vi "Open All Relays_DAQmx_CreateVirtualChannel.vi"(0 "Device/Ports/Lines":string="Dev1/port0/line0,Dev1/port0/line1,Dev1/port0/line2,Dev1/port0/line3,Dev1/port0/line4,Dev1/port0/line5,Dev1/port0/line6,Dev1/port0/line7,\nDev1/port0/line8,Dev1/port0/line9,Dev1/port0/line10,Dev1/port0/line11,Dev1/port0/line12,Dev1/port0/line13,Dev1/port0/line14,Dev1/port0/line15,\nDev1/port0/line16,Dev1/port0/line17,Dev1/port0/line18,Dev1/port0/line19,Dev1/port0/line20,Dev1/port0/line21,\nDev1/port0/line22,Dev1/port0/line23,Dev1/port0/line24,Dev1/port0/line25,\nDev1/port0/line26,Dev1/port0/line27,Dev1/port0/line28,Dev1/port0/line29,Dev1/port0/line30,Dev1/port0/line31,\nDev1/port1/line0,Dev1/port1/line1,Dev1/port1/line2,Dev1/port1/line3,Dev1/port1/line4,Dev1/port1/line5,Dev1/port1/line6,Dev1/port1/line7,\nDev1/port2/line0,Dev1/port2/line1,Dev1/port2/line2,Dev1/port2/line3,Dev1/port2/line4,Dev1/port2/line5,Dev1/port2/line6,Dev1/port2/line7\n", 2 "Boolean":bool, 3 "error in":errorcluster) -> (7 "Array":bool[](array[boolean]), 10 "error out":errorcluster)   [LabVIEW 2015]
uses:
  <vilib>/DAQmx/write.llb/DAQmx Write (Digital 1D Bool 1Chan 1Samp).vi
  <vilib>/DAQmx/create/channels.llb/DAQmx Create Channel (DO-Digital Output).vi
  <vilib>/DAQmx/miscellaneous.llb/DAQmx Fill In Error Info.vi
panel:
  # "False means open relay"
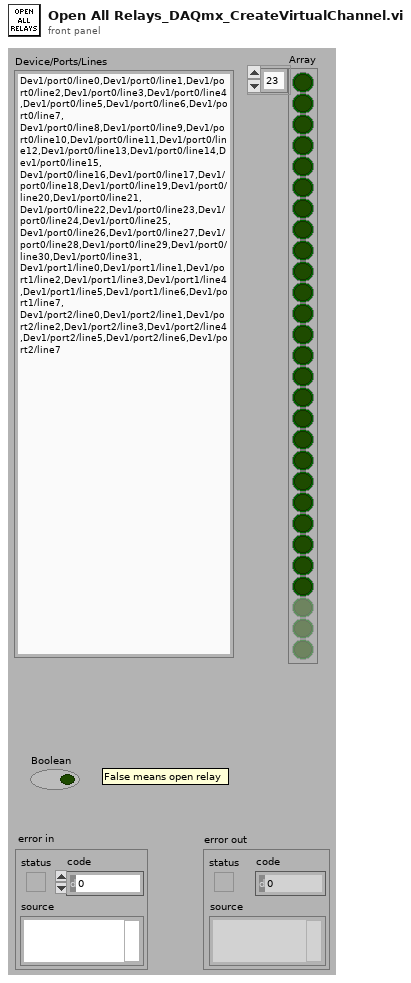
[diagram p1: front panel]
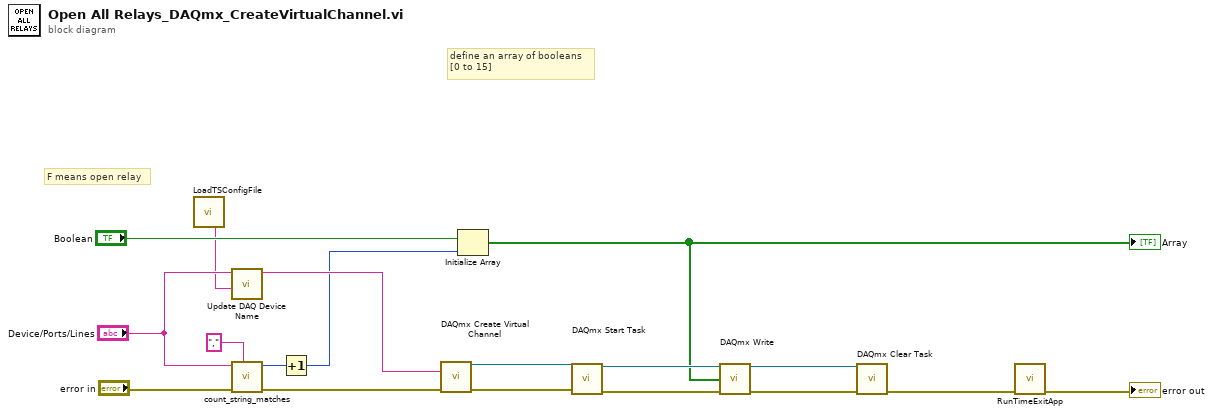
[diagram p0: block diagram]
diagram:
  # "define an array of booleans\n[0 to 15]"
  # "F means open relay"
  n1 = call "LoadTSConfigFile.vi"() -> ("DAQDevice"=w1:string)  [unwired: 5 in, 10 out]
  n2 = call "Update DAQ Device Name.vi"("Device Name"=w1, "Lines in (String)"="Device/Ports/Lines") -> ("Lines out (DAQmx Physical Channels)"=w10:tag)  [unwired: 9 in]
  n3 = call "count_string_matches.vi"("String"="Device/Ports/Lines", "error in (no error)"="error in", "String to Match"=",") -> ("Number of matches"=w18:i32, "error out"=w8:errorcluster)  [unwired: 6 in]
  n4 = Increment(x=w18) -> (x+1=w5:i32)
  n5 = call-poly <vilib>:"DAQmx Create Virtual Channel.vi"("lines"=w10, "error in"=w8) -> ("task out"=w15:refnum<k21>, "error out"=w16:errorcluster)  [unwired: 12 in]
  n6 = Initialize Array("Boolean", w5) -> (w4:bool[])
  "Array" <- w4
  n7 = call <vilib>:"DAQmx Start Task.vi"("task/channels in"=w15, "error in"=w16) -> ("task out"=w14:refnum<k21>, "error out"=w13:errorcluster)  [unwired: 12 in]
  n8 = call-poly <vilib>:"DAQmx Write.vi"("task/channels in"=w14, "data"=w4, "error in"=w13) -> ("task out"=w12:refnum<k21>, "error out"=w11:errorcluster)  [unwired: 10 in, 1 out]
  n9 = call <vilib>:"DAQmx Clear Task.vi"("task in"=w12, "error in"=w11) -> ("error out"=w6:errorcluster)  [unwired: 13 in]
  n10 = call "RunTimeExitApp.vi"("error in (no error)"=w6) -> ("error out"=→"error out":errorcluster)  [unwired: 10 in]
